vi "Basic 4.vi"() -> ()   [LabVIEW 2014, in "Arduino TFT.lvlib"]
uses:
  <vilib>/Aledyne-TSXperts/Arduino Compatible Compiler for LabVIEW/addons/Arduino TFT/Arduino TFT.lvlib
panel:
  out "Error Out":errorcluster
  in  "Error In":errorcluster
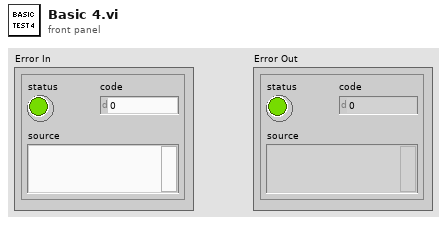
[diagram p1: front panel]
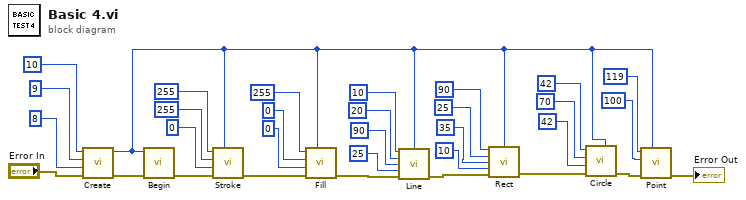
[diagram p0: block diagram]
diagram:
  n1 = call <vilib>:"Create.vi"("Error In"="Error In", "rst"=u8 8 ("cs"), "rs"=u8 9 ("cs"), "cs"=u8 10) -> ("Error Out"=w28:errorcluster, "Instance"=w1:u32)  [unwired: 4 in]
  n2 = call <vilib>:"Begin.vi"("Error In"=w28, "Instance"=w1) -> ("Error Out"=w27:errorcluster)  [unwired: 8 in]
  n3 = call <vilib>:"Stroke.vi"("Instance"=w1, "Error In"=w27, "blue"=u8 0 ("red"), "green"=u8 255 ("red"), "red"=u8 255) -> ("Error Out"=w26:errorcluster)  [unwired: 6 in]
  n4 = call <vilib>:"Fill.vi"("Instance"=w1, "Error In"=w26, "blue"=u8 0 ("red"), "green"=u8 0 ("red"), "red"=u8 255) -> ("Error Out"=w25:errorcluster)  [unwired: 6 in]
  n5 = call <vilib>:"Line.vi"("xStart"=i16 10, "Instance"=w1, "yStart"=i16 20 ("xStart"), "xEnd"=i16 90 ("xStart"), "yEnd"=i16 25 ("xStart"), "Error In"=w25) -> ("Error Out"=w24:errorcluster)  [unwired: 9 in]
  n6 = call <vilib>:"Rect.vi"("x"=i16 90 ("xStart"), "Instance"=w1, "y"=i16 25 ("xStart"), "width"=i16 35 ("xStart"), "height"=i16 10 ("xStart"), "Error In"=w24) -> ("Error Out"=w23:errorcluster)  [unwired: 9 in]
  n7 = call <vilib>:"Circle.vi"("Instance"=w1, "Error In"=w23, "r"=i16 42 ("xStart"), "y"=i16 70 ("xStart"), "x"=i16 42 ("xStart")) -> ("Error Out"=w22:errorcluster)  [unwired: 6 in]
  n8 = call <vilib>:"Point.vi"("Instance"=w1, "Error In"=w22, "y"=u8 100 ("x"), "x"=u8 119) -> ("Error Out"=→"Error Out":errorcluster)  [unwired: 7 in]
